vi "MoAgSy_GPG_writeGpgFiles.vi"(0 "MoAgSy_GPG":refnum<class "MoAgSy_GPG.lvclass">, 5 "error in (no error)":errorcluster) -> (12 "trust db file":path, 14 "dup MoAgSy_GPG":refnum<class "MoAgSy_GPG.lvclass">, 15 "options file":path, 16 "keyring file":path, 17 "sec keyring file":path, 19 "error out":errorcluster)   [LabVIEW 2009, in "MoAgSy.lvlib" / "MoAgSy_GPG.lvclass"]
uses:
  MoAgSy_GPG.lvclass
  MoAgSy_GPG.lvclass/MoAgSy_GPG.ctl
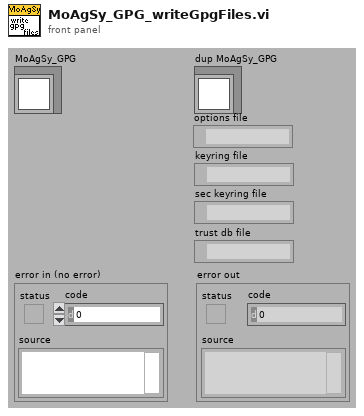
[diagram p1: front panel]
types:
  T1 = cluster{"[0]":path, "[1]":path, "[2]":path, "[3]":path, "[4]":path, "[5]":path, "[6]":path, "[7]":path, "[8]":path}
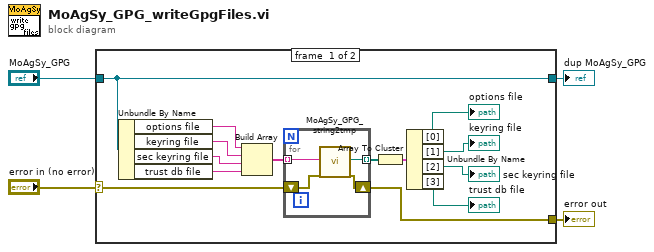
[diagram p0: block diagram]
diagram:
  n1 = case shown="No Error" "error in (no error)" {
    selector: "error in (no error)" -> [w12 w23]
    tunnel: "MoAgSy_GPG" -> [w13 w24]
    tunnel: [w13 w24] -> w3
    tunnel: [w11 w23] -> w1
    frame #0 {
      n2 = Unbundle By Name(w13) -> ("options file"=w18:string, "keyring file"=w17:string, "sec keyring file"=w16:string, "trust db file"=w15:string)
      n3 = Build Array(w18, w17, w16, w15) -> (w14:string[])
      n4 = for {
        tunnel: w14 -> [w22] mode=indexing
        tunnel: [w21] -> w10 mode=indexing
        shift-right: [w19] -> w11
        shift-left: w12 -> [w20]
        n5 = call "MoAgSy_GPG_string2tmp.vi"("String"=w22, "error in (no error)"=w20) -> ("Path"=w21:path, "error out"=w19:errorcluster)  [unwired: 16 out]
      }
      n6 = Array To Cluster(array=w10) -> (cluster=w9:T1)
      n7 = Unbundle By Name(w9) -> ("[0]"=→"options file":path, "[1]"=→"keyring file":path, "[2]"=→"sec keyring file":path, "[3]"=→"trust db file":path)
    }
    frame #1 {
    }
  }
  "dup MoAgSy_GPG" <- w3
  "error out" <- w1
